vi "Untitled 2 (SubVI).vi"(11 "Buttons[8]":bool) -> ()   [LabVIEW 2015]
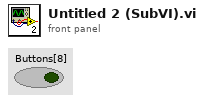
[diagram p1: front panel]
types:
  T1 = typedef "WPI_EncoderDevRef.ctl" = cluster{"DevStatus":errorcluster, "EncoderIndex":T2, "CounterIndex":T3, "DistancePerCount":dbl, "Decoding Type":T4}
  T2 = typedef "FPGA_EncoderIdx.ctl" = enum8{"Enc 0", "Enc 1", "Enc 2", "Enc 3", "Enc 4", "Enc 5", "Enc 6", "Enc 7", "Invalid"}
  T3 = typedef "FPGA_CounterCtrSystemIndex.ctl" = enum8{"Ctr 0", "Ctr 1", "Ctr 2", "Ctr 3", "Ctr 4", "Ctr 5", "Ctr 6", "Ctr 7", "Invalid"}
  T4 = typedef "WPI_EncoderType.ctl" = enum16{"1x", "2x", "4x"}
  T5 = typedef "WPI_PotentiometerDevRef.ctl" = cluster{"DevStatus":errorcluster, "Analog Channel":T6, "Invert Output":bool}
  T6 = typedef "FPGA_AIChannel.ctl" = enum8{"AI 0", "AI 1", "AI 2", "AI 3", "AI MXP 0", "AI MXP 1", "AI MXP 2", "AI MXP 3", "Invalid"}
  T7 = typedef "WPI_MotorControlDeviceRef.ctl" = cluster{"DeviceStatus":errorcluster, "Type":T8, "PWM":cluster{"PWM Channel":T9, "DeadBand":T10}, "CAN":cluster{"Device Number":u8, "Control Mode":T11, "Semaphore":T12, "Max Vout":dbl, "TalonSRX Control Mode":T13}, "Invert":bool}
  T8 = typedef "WPI_MotorControlType.ctl" = enum16{"PWM", "CAN", "CANTalonSRX"}
  T9 = typedef "FPGA_DIOPWMChannel.ctl" = enum8{"PWM 0", "PWM 1", "PWM 2", "PWM 3", "PWM 4", "PWM 5", "PWM 6", "PWM 7", "PWM 8", "PWM 9", "PWM MXP 0", "PWM MXP 1", "PWM MXP 2", "PWM MXP 3", "PWM MXP 4", "PWM MXP 5", "PWM MXP 6", "PWM MXP 7", "PWM MXP 8", "PWM MXP 9", "Invalid"}
  T10 = typedef "WPI_PWMDeadband.ctl" = cluster{"Name":string, "maxPositivePwm":i32, "minPositivePwm":i32, "centerPwm":i32, "maxNegativePwm":i32, "minNegativePwm":i32, "angularRange":u16}
  T11 = typedef "WPI_CANJaguar_ControlMode.ctl" = enum8{"Percent VBus", "Current", "Speed", "Position", "Voltage"}
  T12 = typedef "Semaphore RefNum" = refnum<k1>
  T13 = typedef "WPI_CANTalonSRX_APIControlMode.ctl" = enum8{"Percent VBus", "Speed", "Position", "Slave", "Unchanged / Invalid", "Voltage Compensation", "Current", "Motion Profile"}
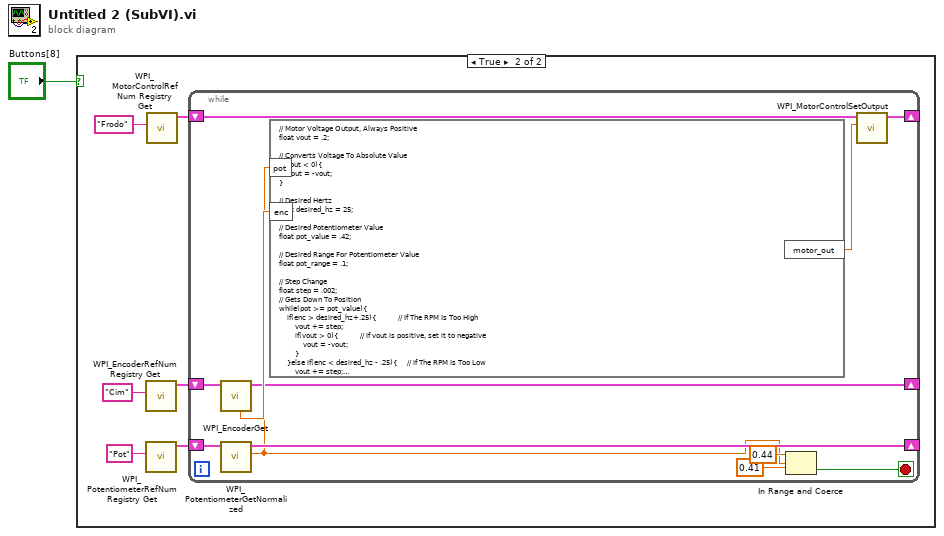
[diagram p0: block diagram]
diagram:
  n1 = case shown="True" "Buttons[8]" {
    frame False {
    }
    frame True {
      n2 = call <vilib>:"WPI_EncoderRefNum Registry Get.vi"("refnum name"="Cim") -> ("EncoderDevRef"=w4:T1)  [unwired: 9 in, 1 out]
      n3 = call <vilib>:"WPI_PotentiometerRefNum Registry Get.vi"("refnum name"="Pot") -> ("PotDevRef"=w7:T5)  [unwired: 9 in, 1 out]
      n4 = call <vilib>:"WPI_MotorControlRefNum Registry Get.vi"("refnum name"="Frodo") -> ("MotorControlDevRef"=w2:T7)  [unwired: 9 in, 1 out]
      n5 = while {
        shift-right: [w18] -> _
        shift-left: w7 -> [w19]
        shift-right: [w15] -> _
        shift-left: w4 -> [w16]
        shift-right: [w12] -> _
        shift-left: w2 -> [w14]
        stop <- w8 stop-if-true
        n6 = call <vilib>:"WPI_EncoderGet.vi"("EncoderDevRef"=w16) -> ("EncoderDevRef"=w15:T1, "Rate"=w17:dbl)  [unwired: 5 in, 4 out]
        n7 = call <vilib>:"WPI_PotentiometerGetNormalized.vi"("PotDevRef"=w19) -> ("Normalized Value"=w9:dbl, "PotDevRef"=w18:T5)  [unwired: 8 in, 1 out]
        n8 = formula code="// Motor Voltage Output, Always Positive\nfloat vout = .2;\n\n// Converts Voltage To Absolute Value\nif(vout < 0){\n    vout = -vout;\n}\n\n// Desired Hertz\nfloat desired_hz = 25;\n\n// Desired Potentiometer Value\nfloat pot_value = .42;\n\n// Desired Range For Potentiometer Value\nfloat pot_range = .1;\n\n// Step Change\nfloat step = .002;\n// Gets Down To Position\nwhile(pot >= pot_value){\n    if(enc > desired_hz+.25){           // If The RPM Is Too High\n        vout += step;\n        if(vout > 0){           // If vout is positive, set it to negative\n            vout = -vout;\n        }\n    }else if(enc < desired_hz - .25){     // If The RPM Is Too Low\n        vout += step; \n        if(vout < 0){           // If vout is negative, set it to positive\n            vout = -vout;\n        }\n    }\n    float motor_out = vout;\n}"("pot"=w9, "enc"=w17) -> ("motor_out"=w13:dbl)
        n9 = In Range and Coerce(upper limit=0.44, x=w9, lower limit=0.41) -> (In Range?=w8:bool)  [unwired: 1 out]
        n10 = call <vilib>:"WPI_MotorControlSetOutput.vi"("Output"=w13, "MotorControlDevRef"=w14) -> ("MotorControlDevRef"=w12:T7)  [unwired: 7 in, 2 out]
      }
    }
  }
